vi "Subscribe to Did Stop.vi"(8 "error in (no error)":errorcluster, 11 "API-Reference in":refnum<data-value>) -> (0 "error out":errorcluster, 2 "Actor Stopped":refnum<event-registration>, 3 "API-Reference out":refnum<data-value>)   [LabVIEW 2018, in "Scripting.lvlib" / "Actor.lvclass"]
uses:
  Actor.lvclass
  API-Data.ctl
  Did Stop.ctl
  Message-Enqueuer References.ctl
  Stop.ctl
  Launch.ctl
  Did Initialize.ctl
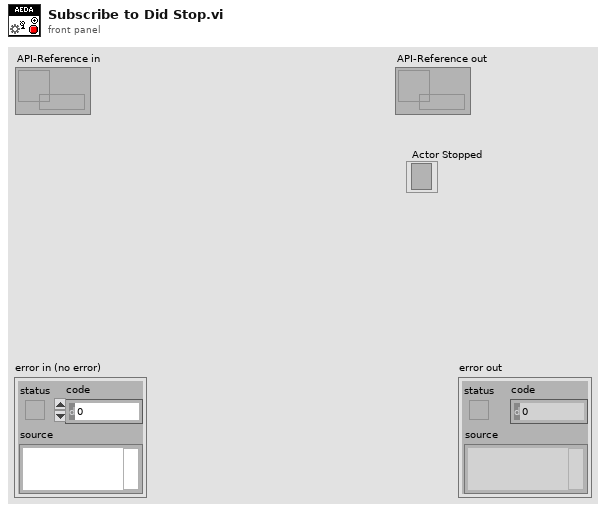
[diagram p1: front panel]
types:
  T1 = typedef "Scripting.lvlib/Actor.lvclass/API-Data.ctl" = cluster{"Launch":refnum<notifier>, "Did Stop Enqueuer":refnum<user-event>, "API":T2, "Did Stop Messages":refnum<event-registration>}
  T2 = typedef "Scripting.lvlib/Actor.lvclass/Message-Enqueuer References.ctl" = cluster{"Stop":refnum<user-event>, "Launch":refnum<user-event>, "Did Initialize":refnum<user-event>}
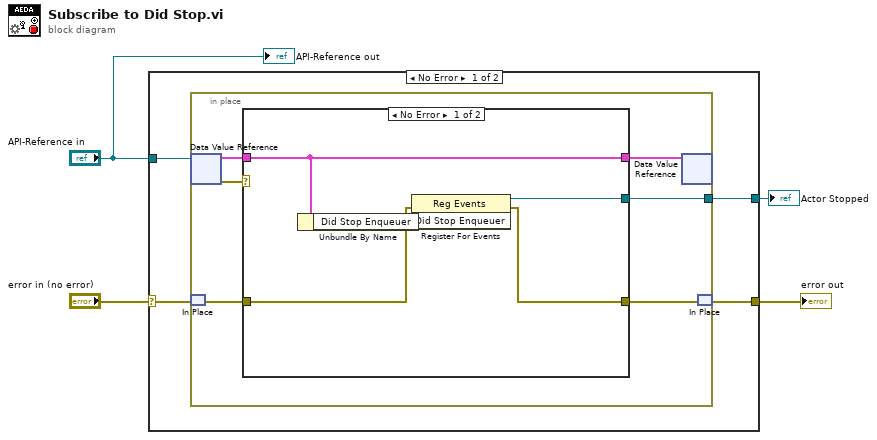
[diagram p0: block diagram]
diagram:
  n1 = case shown="No Error" "error in (no error)" {
    selector: "error in (no error)" -> [w8 w22]
    tunnel: [w7 w22] -> w3
    tunnel: [w6 _] -> w2
    tunnel: "API-Reference in" -> [w5 _]
    frame No Error {
      n2 = in-place {
        in-place-border: [w9] -> w6
        n3 = in-place-dvr #1(w5) -> (w13:T1, w14:errorcluster)
        n4 = in-place-match #2(w8) -> (w11:errorcluster)
        n5 = case shown="No Error" w14 {
          selector: w14 -> [_ w21]
          tunnel: w13 -> [w15 w20]
          tunnel: [w15 w20] -> w12
          tunnel: w11 -> [w19 _]
          tunnel: [w18 w21] -> w10
          tunnel: [w17 _] -> w9
          frame No Error {
            n6 = Unbundle By Name(w15) -> ("Did Stop Enqueuer"=w16:refnum<user-event>)
            n7 = register-events(error in=w19, w16) -> (reference out=w17:refnum<event-registration>, error out=w18:errorcluster)  [unwired: 1 in]
          }
          frame Error {
          }
        }
        n8 = in-place-dvr #1(w12) -> ()  [unwired: 2 out]
        n9 = in-place-match #2(w10) -> (w7:errorcluster)
      }
    }
    frame Error {
    }
  }
  "error out" <- w3
  "Actor Stopped" <- w2
  "API-Reference out" <- "API-Reference in"
